vi "UI-message-definitions.vi"(7 "Message":T2, 8 "error in (no error)":errorcluster, 10 "Additional text":string, 11 "ModComm in":T1) -> (0 "error out":errorcluster, 3 "ModComm out":T1)   [LabVIEW 2013, in "Server.lvlib" / "Server.lvclass"]
uses:
  Server.lvclass
  UI-messages.ctl
  Object-reference.ctl
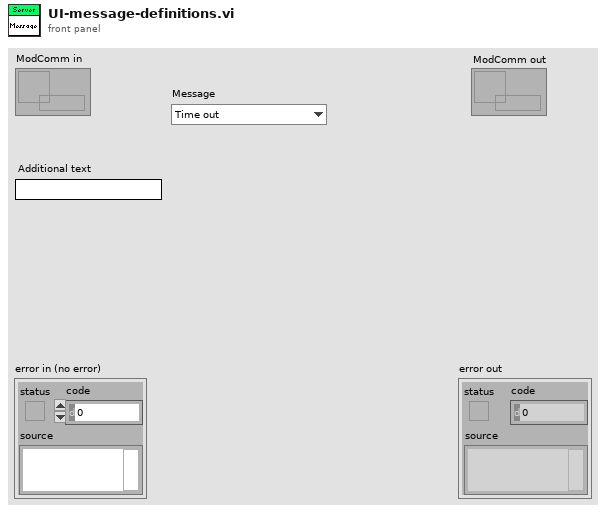
[diagram p1: front panel]
types:
  T1 = typedef "Server.lvlib/Server.lvclass/Object-reference.ctl" = refnum<data-value>
  T2 = typedef "Server.lvlib/Server.lvclass/UI-messages.ctl" = enum16{"Time out", "User cancel", "Module cancel", "Client inactivity", "Client limit", "Client started"}
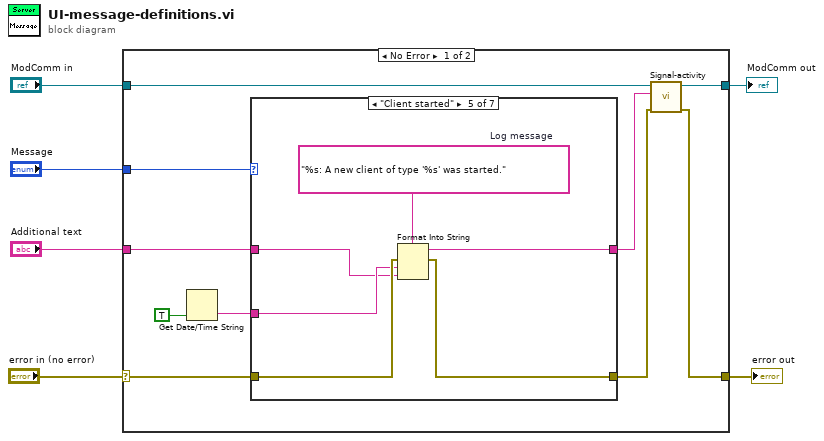
[diagram p0: block diagram]
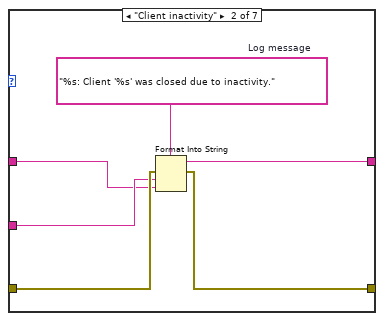
[diagram p3: hidden frame]
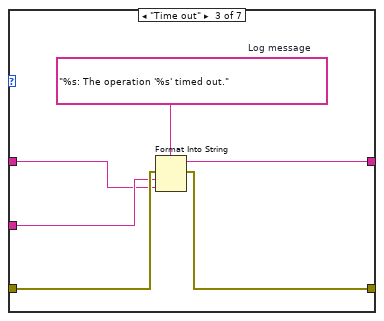
[diagram p4: hidden frame]
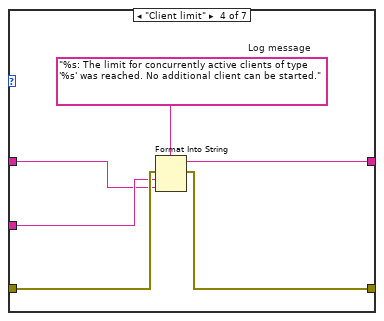
[diagram p5: hidden frame]
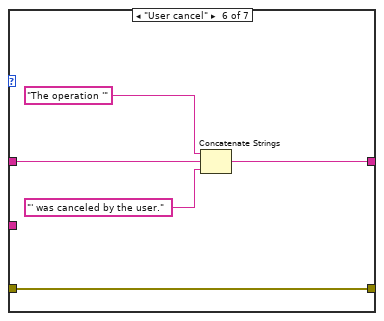
[diagram p6: hidden frame]
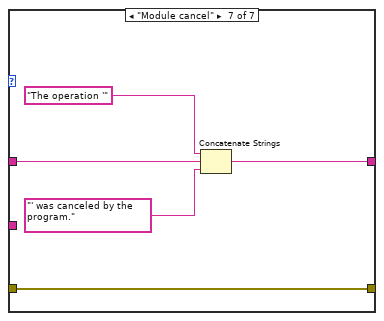
[diagram p7: hidden frame]
diagram:
  n1 = case shown="No Error" "error in (no error)" {
    selector: "error in (no error)" -> [w16 w53]
    tunnel: [w11 w53] -> w5
    tunnel: "Message" -> [w15 _]
    tunnel: "Additional text" -> [w14 _]
    tunnel: "ModComm in" -> [w13 w52]
    tunnel: [w12 w52] -> w2
    frame No Error {
      n2 = Get Date/Time String(want seconds? (F)=TRUE) -> (time string=w8:string)  [unwired: 2 in, 1 out]
      n3 = case shown="\"Client started\"" w15 {
        tunnel: w16 -> [w17 w21 w27 w33 w39 w46 w51]
        tunnel: w14 -> [_ w18 w24 w30 w36 w45 w50]
        tunnel: [w17 w20 w26 w32 w38 w46 w51] -> w10
        tunnel: [_ w22 w28 w34 w40 w42 w47] -> w9
        tunnel: w8 -> [_ w19 w25 w31 w37 _ _]
        frame Default {
        }
        frame "Client inactivity" {
          w23 = "%s: Client '%s' was closed due to inactivity."  # Log message
          n4 = Format Into String(format string=w23, error in=w21, w19, w18) -> (resulting string=w22:string, error out=w20:errorcluster)  [unwired: 1 in]
        }
        frame "Time out" {
          w29 = "%s: The operation '%s' timed out."  # Log message
          n5 = Format Into String(format string=w29, error in=w27, w25, w24) -> (resulting string=w28:string, error out=w26:errorcluster)  [unwired: 1 in]
        }
        frame "Client limit" {
          w35 = "%s: The limit for concurrently active clients of type '%s' was reached. No additional client can be started."  # Log message
          n6 = Format Into String(format string=w35, error in=w33, w31, w30) -> (resulting string=w34:string, error out=w32:errorcluster)  [unwired: 1 in]
        }
        frame "Client started" {
          w41 = "%s: A new client of type '%s' was started."  # Log message
          n7 = Format Into String(format string=w41, error in=w39, w37, w36) -> (resulting string=w40:string, error out=w38:errorcluster)  [unwired: 1 in]
        }
        frame "User cancel" {
          n8 = Concatenate Strings("The operation '", w45, "' was canceled by the user.") -> (w42:string)
        }
        frame "Module cancel" {
          n9 = Concatenate Strings("The operation '", w50, "' was canceled by the program.") -> (w47:string)
        }
      }
      n10 = call "Signal-activity.vi"("error in (no error)"=w10, "Log message"=w9, "ModComm in"=w13) -> ("error out"=w11:errorcluster, "ModComm out"=w12:T1)  [unwired: 7 in]
    }
    frame Error {
    }
  }
  "error out" <- w5
  "ModComm out" <- w2
